vi "Extract Data from Menu Ref.vi"(8 "error in (no error)":errorcluster, 9 "Starting Tag":string, 10 "Menu Items in":T2(array[cluster]), 11 "menu reference":refnum<k9>) -> (0 "error out":errorcluster, 2 "Menu Items out":T2(array[cluster]), 3 "menu reference out":refnum<k9>)   [LabVIEW 2013, in "SET Project Data.lvlib" / "Menu Data.lvclass"]
uses:
  Menu Data.lvclass
  <vilib>/Utility/miscctls.llb/LVMenuShortCut.ctl
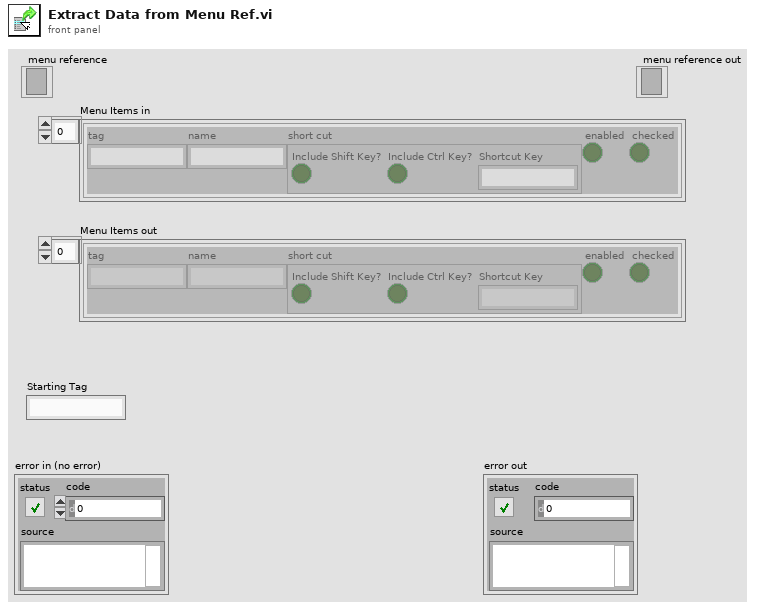
[diagram p1: front panel]
types:
  T1 = typedef "LVMenuShortCut.ctl" = cluster{"Include Shift Key?":bool, "Include Ctrl Key?":bool, "Shortcut Key":string}
  T2 = cluster{"tag":string, "name":string, "short cut":T1, "enabled":bool, "checked":bool}[]
  T3 = cluster{"tag":string, "name":string, "short cut":T1, "enabled":bool, "checked":bool}
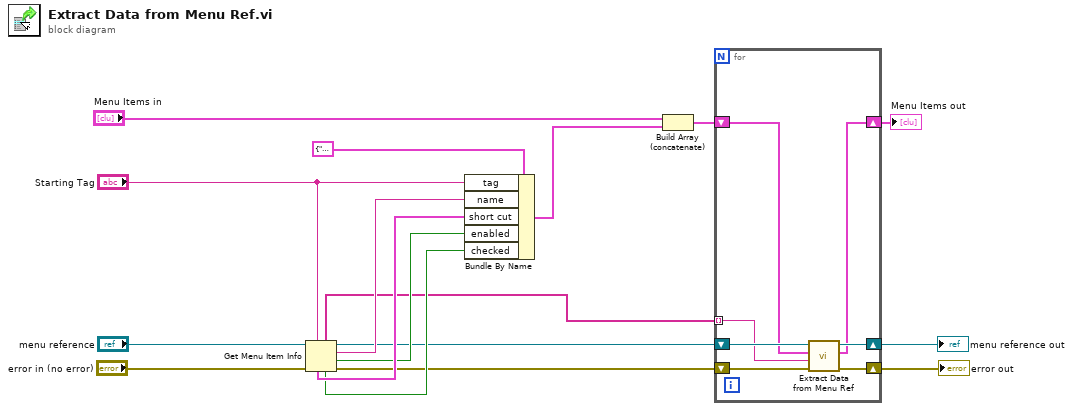
[diagram p0: block diagram]
diagram:
  n1 = Get Menu Item Info(7:"Starting Tag", 8:"error in (no error)", 11:"menu reference") -> (0:w6:errorcluster, 1:w10:bool, 2:w12:string, 3:w7:refnum<k9>, 4:w9:bool, 5:w1:string[], 6:w11:T1)
  n2 = Bundle By Name(cluster=T3 {"tag"="", "name"="", "short cut"={"Include Shift Key?"=FALSE, "Include Ctrl Key?"=FALSE, "Shortcut Key"=""}, "enabled"=FALSE, "checked"=FALSE}, "tag"="Starting Tag", "name"=w12, "short cut"=w11, "enabled"=w10, "checked"=w9) -> (w8:T3)
  n3 = Build Array (concatenate)("Menu Items in", w8) -> (w5:T2)
  n4 = for {
    tunnel: w1 -> [w20] mode=indexing
    shift-right: [w23] -> w2
    shift-left: w7 -> [w24]
    shift-right: [w21] -> w3
    shift-left: w6 -> [w22]
    shift-right: [w18] -> w4
    shift-left: w5 -> [w19]
    n5 = call "Extract Data from Menu Ref.vi"("error in (no error)"=w22, "Starting Tag"=w20, "Menu Items in"=w19, "menu reference"=w24) -> ("error out"=w21:errorcluster, "Menu Items out"=w18:T2, "menu reference out"=w23:refnum<k9>)  [unwired: 5 in]
  }
  "menu reference out" <- w2
  "error out" <- w3
  "Menu Items out" <- w4
